vi "Teleop.vi"(10 "Match Info":T2={"Autonomous Elapsed Seconds"=0.0, "TeleOp Elapsed Seconds"=0.0, "Disabled Elapsed Seconds"=0.0, "Visited Autonomous"=FALSE, "Visited TeleOp"=FALSE, "Visited Disabled"=FALSE, "Autonomous Settings"={"Autonomous Style"=enum."Independent", "VI Refnum"=refnum}}, 11 "Call Context":T3) -> ()   [LabVIEW 2014]
doc: "This VI is called for each TeleOp packet received from the DS where the robot is not disabled. It is often used to read from the joysticks and update I/O or to update setpoints for timed control loops. It should complete and return within 20 milliseconds or it may miss DS packets."
uses:
  <vilib>/Rock Robotics/WPI/DriverStation/WPI_DriverStationDerivedRobotMode.ctl
  <vilib>/Rock Robotics/WPI/DriverStation/WPI_DriverStationMatch Info.ctl
  <vilib>/Rock Robotics/WPI/Ultrasonic/WPI_UltrasonicRangeUnits.ctl
  <vilib>/Rock Robotics/WPI/Joystick/WPI_JoystickGetSetRefNum.vi
  <vilib>/Rock Robotics/Network Tables/SD Write Boolean Array.vi
  <vilib>/Rock Robotics/Network Tables/SD Write Numeric Array.vi
  <vilib>/Rock Robotics/Network Tables/SD Read Boolean.vi
  <vilib>/Rock Robotics/Network Tables/SD Read Number.vi
  <vilib>/Rock Robotics/WPI/Ultrasonic/WPI_SonarSRF04DigitalRefNum Registry Get.vi
  <vilib>/Rock Robotics/WPI/Ultrasonic/WPI_SonarSRF04DigitalGetRange.vi
  <vilib>/Rock Robotics/WPI/Solenoid/Deprecated/WPI_SolenoidSetBool.vi
  <vilib>/Rock Robotics/WPI/Solenoid/WPI_SolenoidGetEnum.vi
panel:
  in  "Intake PID gains":T1={"proportional gain (Kc)"=1.0, "integral time (Ti, min)"=0.01, "derivative time (Td, min)"=0.0} {"derivative time (Td, min)" format="%.3f"; "integral time (Ti, min)" format="%.3f"; "proportional gain (Kc)" format="%.3f"}
  in  "PID gains Fast":T1={"proportional gain (Kc)"=0.7500000000000001, "integral time (Ti, min)"=0.001, "derivative time (Td, min)"=0.0} {"derivative time (Td, min)" format="%.3f"; "integral time (Ti, min)" format="%.3f"; "proportional gain (Kc)" format="%.3f"}
  in  "Lift PID gains":T1={"proportional gain (Kc)"=1.0, "integral time (Ti, min)"=0.01, "derivative time (Td, min)"=0.0} {"derivative time (Td, min)" format="%.3f"; "integral time (Ti, min)" format="%.3f"; "proportional gain (Kc)" format="%.3f"}
  out "Distance?":bool
  out "Distance":dbl
  in  "PID gains Slow":T1={"proportional gain (Kc)"=0.7500000000000001, "integral time (Ti, min)"=0.004, "derivative time (Td, min)"=0.0} {"derivative time (Td, min)" format="%.3f"; "integral time (Ti, min)" format="%.3f"; "proportional gain (Kc)" format="%.3f"}
  out "XY Graph":cluster{dbl[], dbl[]}(graph)
  out "Z Axis max":dbl
  out "Solenoid true":bool
  out "Y Axis max":dbl
  out "X Axis max":dbl
  in  "H Tank Disabled":bool
  out "Sample Slider 0":dbl(slide) scale=0.0..5.0
  out "Sample Boolean 1":bool
  out "Sample Boolean 0":bool
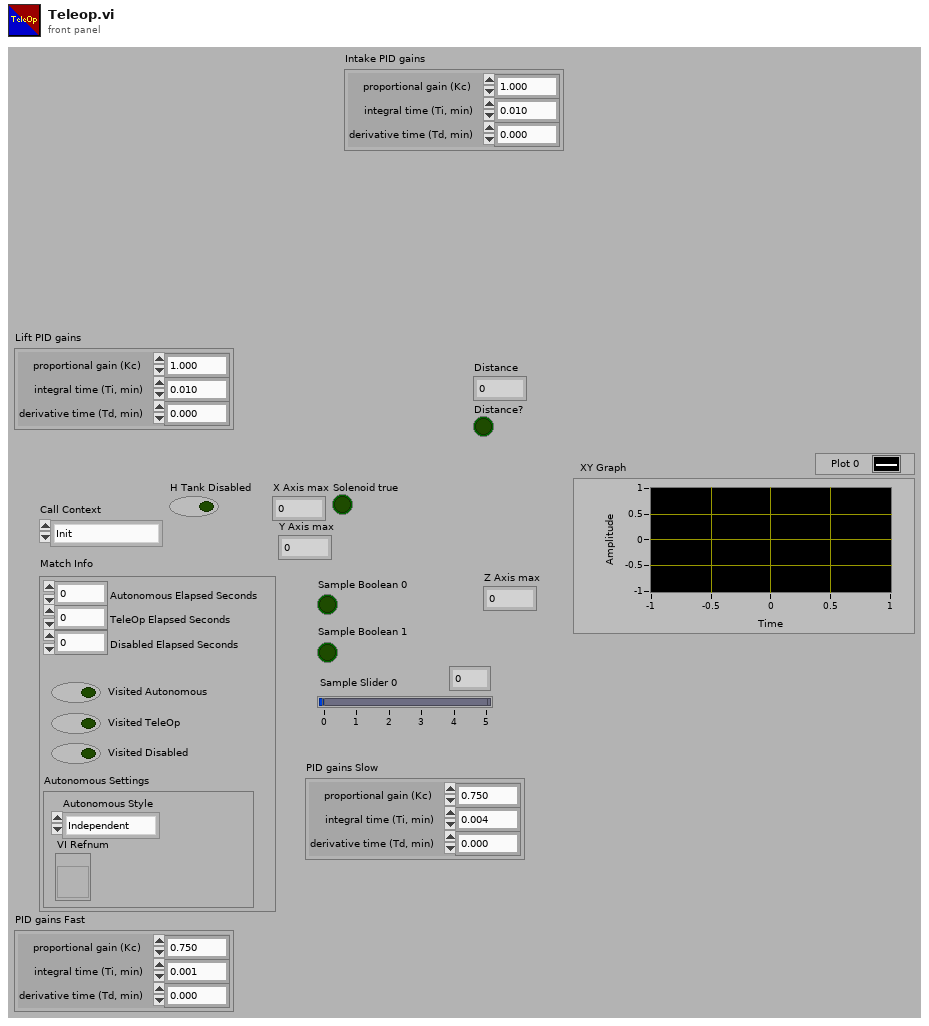
[diagram p1: front panel]
types:
  T1 = cluster{"proportional gain (Kc)":dbl, "integral time (Ti, min)":dbl, "derivative time (Td, min)":dbl}
  T2 = typedef "WPI_DriverStationMatch Info.ctl" = cluster{"Autonomous Elapsed Seconds":dbl, "TeleOp Elapsed Seconds":dbl, "Disabled Elapsed Seconds":dbl, "Visited Autonomous":bool, "Visited TeleOp":bool, "Visited Disabled":bool, "Autonomous Settings":cluster{"Autonomous Style":enum16{"Iterative", "Independent"}, "VI Refnum":refnum<vi>}}
  T3 = typedef "WPI_DriverStationDerivedRobotMode.ctl" = enum16{"Init", "Execute", "Stop"}
  T4 = typedef "WPI_UltrasonicRangeUnits.ctl" = enum16{"inches", "mm"}
  T5 = typedef "WPI_JoystickDevRef.ctl" = cluster{"Device":T6}
  T6 = typedef "WPI_JoystickDeviceEnum.ctl" = enum16{"USB 0", "USB 1", "USB 2", "USB 3", "USB 4", "USB 5"}
  T7 = typedef "WPI_UltrasonicDeviceRef.ctl" = cluster{"DevStatus":errorcluster, "Ping Digital Controller":T8, "Echo Digital Controller":T8, "Ping Channel":T9, "Echo Channel":T9, "CntIndex":T10}
  T8 = typedef "FPGA_TypedefDigitalModule.ctl" = enum16{"Controller 1"}
  T9 = typedef "FPGA_DIOChannel.ctl" = enum8{"DIO 0", "DIO 1", "DIO 2", "DIO 3", "DIO 4", "DIO 5", "DIO 6", "DIO 7", "DIO 8", "DIO 9", "DIO MXP 0", "DIO MXP 1", "DIO MXP 2", "DIO MXP 3", "DIO MXP 4", "DIO MXP 5", "DIO MXP 6", "DIO MXP 7", "DIO MXP 8", "DIO MXP 9", "DIO MXP 10", "DIO MXP 11", "DIO MXP 12", "DIO MXP 13", "DIO MXP 14", "DIO MXP 15", "Invalid"}
  T10 = typedef "FPGA_CounterCtrSystemIndex.ctl" = enum8{"Ctr 0", "Ctr 1", "Ctr 2", "Ctr 3", "Ctr 4", "Ctr 5", "Ctr 6", "Ctr 7", "Invalid"}
  T11 = typedef "WPI_EncoderDevRef.ctl" = cluster{"DevStatus":errorcluster, "EncoderIndex":T12, "CounterIndex":T10, "DistancePerCount":dbl, "Decoding Type":T13}
  T12 = typedef "FPGA_EncoderIdx.ctl" = enum8{"Enc 0", "Enc 1", "Enc 2", "Enc 3", "Enc 4", "Enc 5", "Enc 6", "Enc 7", "Invalid"}
  T13 = typedef "WPI_EncoderType.ctl" = enum16{"1x", "2x", "4x"}
  T14 = typedef "WPI_AccelerometerDevRef.ctl" = cluster{"DevStatus":errorcluster, "Controller":T15, "Scaling":T16, "Analog Channels":T17, "I2C Bus":T19, "SPI Bus":T20, "Accel Range":T21, "ADXL345 Axes":T22, "Handle":i32, "Device Address":u8, "Accel Type":enum16{"Analog", "ADXL345 I2C", "ADXL345 SPI", "Internal"}}
  T15 = typedef "FPGA_TypedefAnalogModule.ctl" = enum16{"Controller 1"}
  T16 = typedef "WPI_AccelerometerScaling.ctl" = cluster{"Gain (VoltsPerG)":dbl, "Center Voltage":dbl}
  T17 = typedef "WPI_AccelerometerAnalogChannels.ctl" = cluster{"X-Axis":T18, "Y-Axis":T18, "Z-Axis":T18}
  T18 = typedef "FPGA_AIChannel.ctl" = enum8{"AI 0", "AI 1", "AI 2", "AI 3", "AI MXP 0", "AI MXP 1", "AI MXP 2", "AI MXP 3", "Invalid"}
  T19 = typedef "i2c_bus.ctl" = enum16{"I2C On-Board", "I2C MXP", "Invalid"}
  T20 = typedef "spi_bus.ctl" = enum16{"SPI On-Board, CS0", "SPI On-Board, CS1", "SPI On-Board, CS2", "SPI On-Board, CS3", "SPI MXP", "Invalid"}
  T21 = typedef "ADXL345 Range.ctl" = u8
  T22 = typedef "WPI_AccelerometerADXL345 Axes.ctl" = cluster{"X-Axis":bool, "Y-Axis":bool, "Z-Axis":bool}
  T23 = cluster{"X-Axis":dbl, "Y-Axis":dbl, "Z-Axis":dbl}
  T24 = typedef "WPI_SolenoidDevRef.ctl" = cluster{"DevStatus":errorcluster, "Pneumatics Control Module":u8, "Forward Solenoid Channel":T25, "Reverse Solenoid Channel":T25}
  T25 = typedef "WPI_SolenoidChannel.ctl" = enum8{"Solenoid 0", "Solenoid 1", "Solenoid 2", "Solenoid 3", "Solenoid 4", "Solenoid 5", "Solenoid 6", "Solenoid 7", "Invalid"}
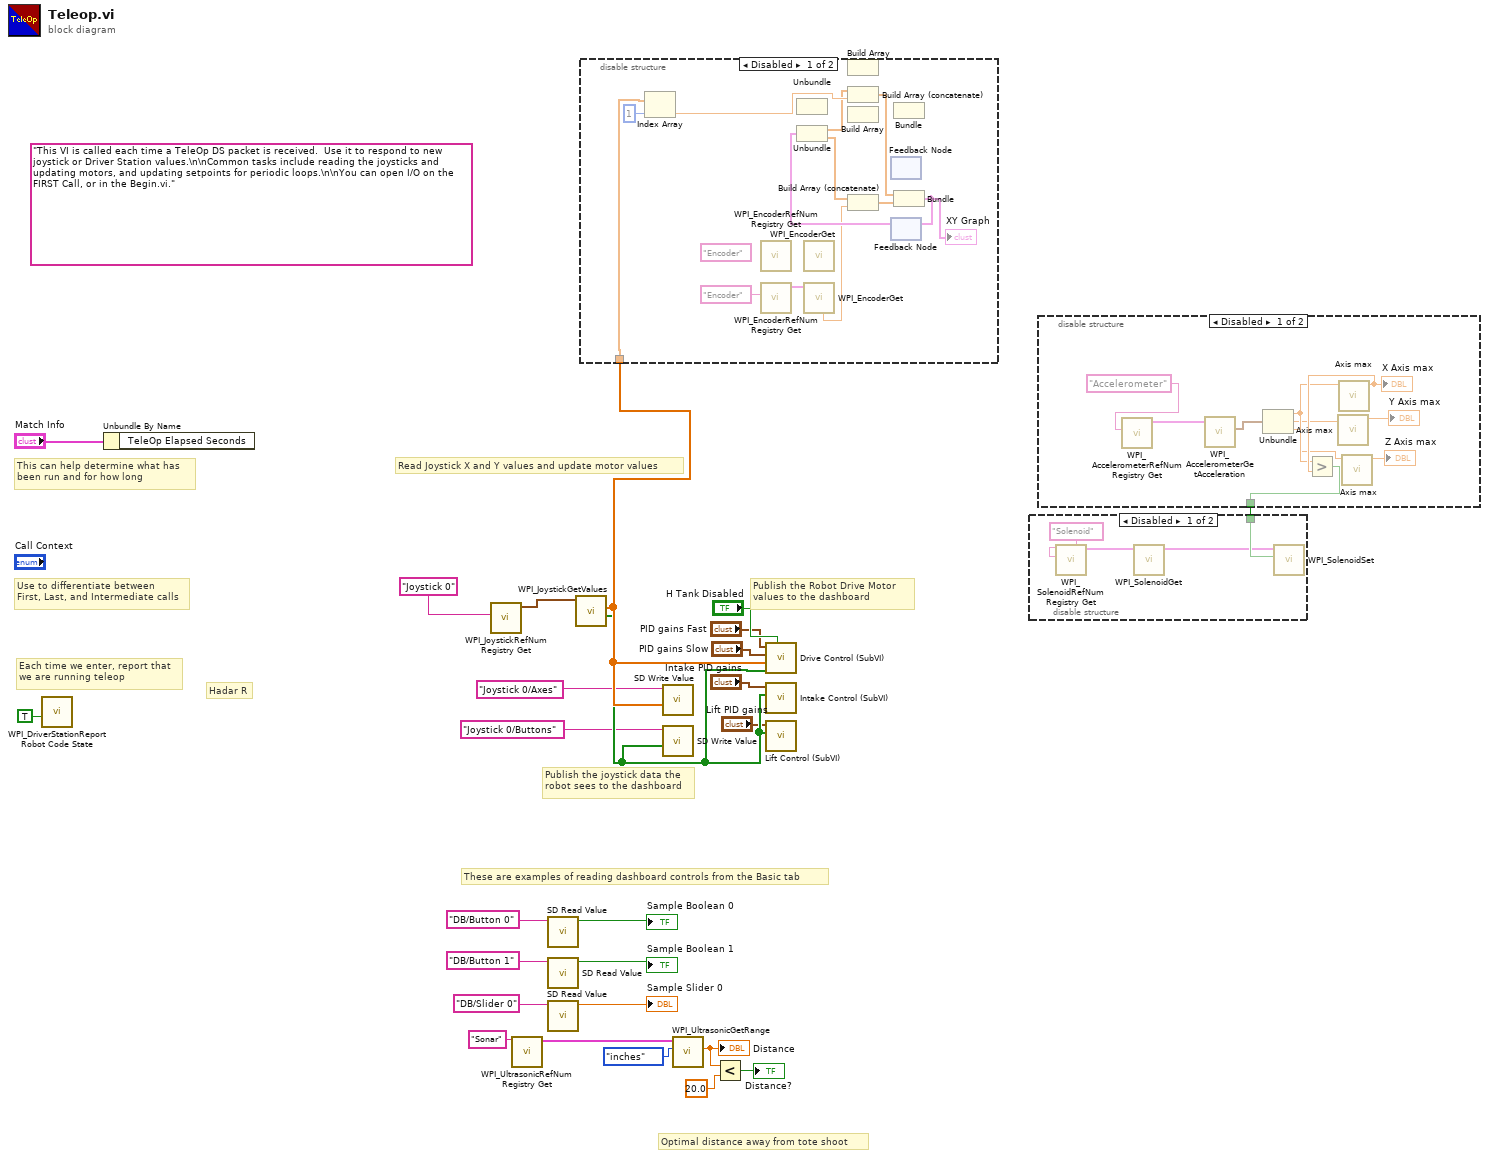
[diagram p0: block diagram]
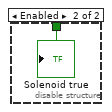
[diagram p3: hidden frame]
diagram:
  (unwired) "This VI is called each time a TeleOp DS packet is received.  Use it to respond to new joystick or Driver Station values.\n\nCommon tasks include reading the joysticks and updating motors, and updating setpoints for periodic loops.\n\nYou can open I/O on the FIRST Call, or in the Begin.vi."
  # "Hadar R"
  # "Optimal distance away from tote shoot"
  # "These are examples of reading dashboard controls from the Basic tab"
  # "Publish the Robot Drive Motor\nvalues to the dashboard"
  # "Publish the joystick data the\nrobot sees to the dashboard"
  # "Each time we enter, report that\nwe are running teleop"
  # "Use to differentiate between\nFirst, Last, and Intermediate calls"
  # "This can help determine what has\nbeen run and for how long"
  # "Read Joystick X and Y values and update motor values"
  n1 = call <vilib>:"WPI_DriverStationReport Robot Code State.vi"("TeleOp"=TRUE ("Autonomous")) -> ()  [unwired: 10 in, 1 out]
  n2 = Unbundle By Name("Match Info") -> ()  [unwired: 1 out]
  n3 = call <vilib>:"WPI_JoystickRefNum Registry Get.vi"("refnum name"="Joystick 0") -> ("JoystickDevRef"=w24:T5)  [unwired: 1 in, 9 out]
  n4 = call-poly <vilib>:"WPI_UltrasonicRefNum Registry Get.vi"("refnum name"="Sonar") -> ("SonarSRF04DevRef"=w5:T7)  [unwired: 9 in, 1 out]
  n5 = call-poly <vilib>:"SD Read Value.vi"("Name"="DB/Button 0" ("refnum name")) -> ("Boolean"=→"Sample Boolean 0":bool)  [unwired: 8 in, 2 out]
  n6 = call-poly <vilib>:"SD Read Value.vi"("Name"="DB/Button 1" ("refnum name")) -> ("Boolean"=→"Sample Boolean 1":bool)  [unwired: 8 in, 2 out]
  n7 = call-poly <vilib>:"SD Read Value.vi"("Name"="DB/Slider 0" ("refnum name")) -> ("Numeric"=→"Sample Slider 0":dbl)  [unwired: 8 in, 2 out]
  n8 = call <vilib>:"WPI_JoystickGetValues.vi"("JoystickDevRef"=w24) -> ("Buttons"=w16:bool[], "Axes"=w18:dbl[])  [unwired: 6 in, 3 out]
  n9 = disable-structure shown="Disabled" {
    disable-tunnel: w18 -> [w38 _]
    frame Disabled {
      (unwired) "Encoder" ("refnum name")
      n10 = Index Array(array=w38, index=1) -> (element=w37:dbl)
      n11 = call <vilib>:"WPI_EncoderRefNum Registry Get.vi"() -> ()  [unwired: 10 in, 2 out]
      n12 = call <vilib>:"WPI_EncoderRefNum Registry Get.vi"("refnum name"="Encoder") -> ("EncoderDevRef"=w28:T11)  [unwired: 9 in, 1 out]
      n13 = Unbundle() -> ()  [unwired: 1 in, 2 out]
      n14 = call <vilib>:"WPI_EncoderGet.vi"() -> ()  [unwired: 6 in, 6 out]
      n15 = call <vilib>:"WPI_EncoderGet.vi"("EncoderDevRef"=w28) -> ("Rate"=w29:dbl)  [unwired: 5 in, 5 out]
      n16 = Build Array() -> ()  [unwired: 2 in, 1 out]
      n17 = Build Array() -> ()  [unwired: 2 in, 1 out]
      n18 = feedback #1() -> ()  [unwired: 2 in]
      n19 = feedback-in #1() -> ()  [unwired: 1 out]
      n20 = feedback #2() -> (w32:cluster{dbl[], dbl[]})  [unwired: 1 in]
      n21 = Unbundle(w32) -> (w34:dbl[], w33:dbl[])
      n22 = Build Array (concatenate)(w34, w37) -> (w35:dbl[])
      n23 = Build Array (concatenate)(w33, w29) -> (w30:dbl[])
      n24 = Bundle() -> ()  [unwired: 3 in, 1 out]
      n25 = Bundle(w35, w30) -> (w31:cluster{dbl[], dbl[]})  [unwired: 1 in]
      "XY Graph" <- w31
      n26 = feedback-in #2(w31) -> ()
    }
    frame Enabled {
    }
  }
  n27 = call-poly <vilib>:"SD Write Value.vi"("Numeric Array"=w18, "Name"="Joystick 0/Axes") -> ()  [unwired: 8 in, 2 out]
  n28 = call-poly <vilib>:"SD Write Value.vi"("Boolean Array"=w16, "Name"="Joystick 0/Buttons") -> ()  [unwired: 8 in, 2 out]
  n29 = call-poly <vilib>:"WPI_UltrasonicGetRange.vi"("Range Units"=WPI_UltrasonicRangeUnits."inches", "UltrasonicDevRef"=w5) -> ("Distance"=w4:dbl)  [unwired: 7 in, 2 out]
  "Distance" <- w4
  n30 = Less?(x=w4, y=20.0) -> (x < y?=→"Distance?":bool)
  n31 = call "Drive Control (SubVI).vi"("H Tank Disabled"="H Tank Disabled", "Buttons"=w16, "Joystick Axis"=w18, "PID gains Slow"="PID gains Slow", "PID gains Fast"="PID gains Fast") -> ()  [unwired: 7 in]
  n32 = call "Intake Control (SubVI).vi"("Buttons"=w16, "Intake PID gains"="Intake PID gains") -> ()  [unwired: 10 in]
  n33 = call "Lift Control (SubVI).vi"("Buttons"=w16, "Lift PID gains"="Lift PID gains") -> ()  [unwired: 10 in]
  n34 = disable-structure shown="Disabled" {
    disable-tunnel: [w48 _] -> w7
    frame Disabled {
      n35 = call <vilib>:"WPI_AccelerometerRefNum Registry Get.vi"("refnum name"="Accelerometer") -> ("AccelerometerDevRef"=w42:T14)  [unwired: 9 in, 1 out]
      n36 = call <vilib>:"WPI_AccelerometerGetAcceleration.vi"("AccelerometerDevRef"=w42) -> ("Accelerations"=w43:T23)  [unwired: 8 in, 2 out]
      n37 = Unbundle(w43) -> ("X-Axis"=w46:dbl, "Y-Axis"=w45:dbl, "Z-Axis"=w44:dbl)
      n38 = call "Axis max.vi"("Axis"=w45) -> ("Axis max"=→"Y Axis max":dbl)  [unwired: 10 in]
      n39 = call "Axis max.vi"("Axis"=w46) -> ("Axis max"=w47:dbl)  [unwired: 10 in]
      "X Axis max" <- w47
      n40 = Greater?(x=w46, y=w47) -> (0:w48:bool)
      n41 = call "Axis max.vi"("Axis"=w44) -> ("Axis max"=→"Z Axis max":dbl)  [unwired: 10 in]
    }
    frame Enabled {
    }
  }
  n42 = disable-structure shown="Disabled" {
    disable-tunnel: w7 -> [w52 w53]
    frame Disabled {
      n43 = call <vilib>:"WPI_SolenoidRefNum Registry Get.vi"("refnum name"="Solenoid") -> ("SolenoidDevRef"=w50:T24)  [unwired: 9 in, 1 out]
      n44 = call-poly <vilib>:"WPI_SolenoidGet.vi"("SolenoidDevRef"=w50) -> ("SolenoidDevRef"=w51:T24)  [unwired: 8 in, 2 out]
      n45 = call-poly <vilib>:"WPI_SolenoidSet.vi"("Value"=w52, "SolenoidDevRef"=w51) -> ()  [unwired: 8 in, 2 out]
    }
    frame Enabled {
      "Solenoid true" <- w53
    }
  }
